vi "S1500_S7Com_W+R_Loop.vi"() -> ()   [LabVIEW 2018]
doc: "Demonstrates Reading from and Writing to a PLC in a loop."
uses:
  S7Com_Source_inkl_IP/S7Com_PLC_Data.ctl
  S1500_S7Com_Data_Array.ctl
  S1500_S7Com_RW_CMD.ctl
  S1500_S7Com_Address_Area.ctl
  S1500_S7Com_Start_Add.ctl
  S1500_S7Com_Transport_Size.ctl
  S1500_S7Com_Function.ctl
  S7Com_Source_inkl_IP/S7Com_Function.ctl
  S7Com_Source_inkl_IP/S7Com_Transport_Size.ctl
  S7Com_Source_inkl_IP/S7Com_Address_Area.ctl
  S7Com_Source_inkl_IP/S7Com_Start_Add.ctl
  S7Com_Source_inkl_IP/S7Com_RW_CMD.ctl
panel:
  out "x+1":u32
  out "Read_Data 2":T1
  in  "RW_CMD":T2={"Read Length"=1, "Data Block #"=1, "S7_Add_Area"=132, "Start Address"=0, "S7_Transport_Size"=5, "S7_Function"=2, "IP-Address"=""} {"S7_Function" items=["Read"=4, "Write"=5]; "S7_Transport_Size" items=["BIT"=1, "BYTE"=2, "CHAR"=3, "WORD"=4, "INT"=5, "DWORD"=6, "DINT"=7, "REAL"=8]; "S7_Add_Area" items=["P Area"=128, "I Area"=129, "O Area"=130, "M Area"=131, "DB Area"=132, "Counter"=40, "Timer"=41]}
  out "Read_Data":T1
  out "Loops":u32
  out "Data from PLC":T7
  in  "Data to PLC":T7
  out "Write Error":bool
  out "Read Error":bool=TRUE
  in  "wait":u32=1000 min=500 step=1
  in  "stop":bool
  in  "timeout ms":i32=5000
  in  "PLC IP Address":string="192.168.84.1"
  out "error out":errorcluster={"status"=TRUE, "code"=59, "source"="LIB_PLC_communication.lvlib:S1500_S7Com_OPEN(SubVI).vi:6290002->LIB_PLC_communication.lvlib:S1500_S7Com_W+R_Loop.vi中的打开TCP连接"}
  in  "error in (no error)":errorcluster
  # "DB-12, Write to PLC"
  # "DB-11, Read from PLC"
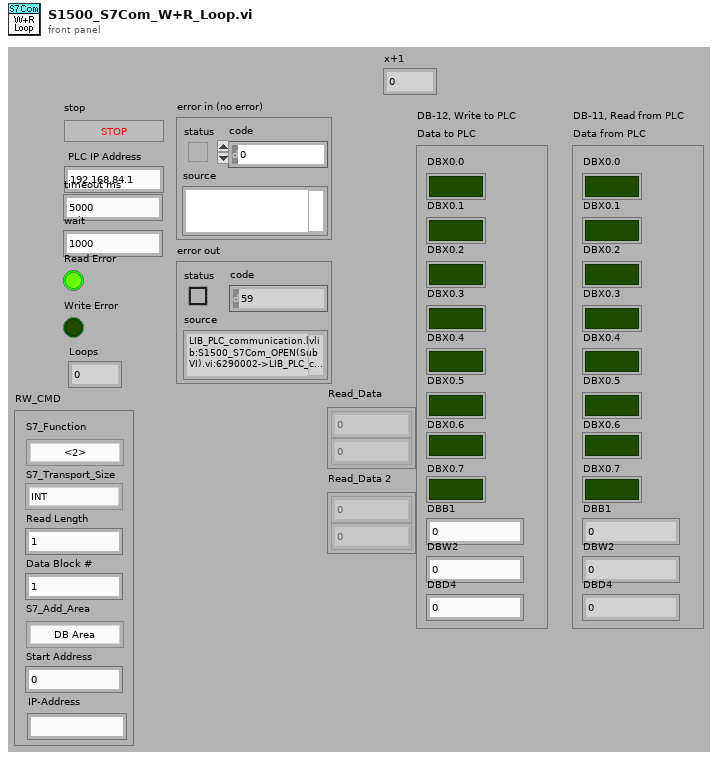
[diagram p1: front panel]
types:
  T1 = typedef "S1500_S7Com_Data_Array.ctl" = i32[]
  T2 = typedef "S1500_S7Com_RW_CMD.ctl" = cluster{"Read Length":u16, "Data Block #":u16, "S7_Add_Area":T3, "Start Address":T4, "S7_Transport_Size":T5, "S7_Function":T6, "IP-Address":string}
  T3 = typedef "S1500_S7Com_Address_Area.ctl" = u8
  T4 = typedef "S1500_S7Com_Start_Add.ctl" = u16
  T5 = typedef "S1500_S7Com_Transport_Size.ctl" = u8
  T6 = typedef "S1500_S7Com_Function.ctl" = u8
  T7 = typedef "S7Com_PLC_Data.ctl" = cluster{"DBX0.0":bool, "DBX0.1":bool, "DBX0.2":bool, "DBX0.3":bool, "DBX0.4":bool, "DBX0.5":bool, "DBX0.6":bool, "DBX0.7":bool, "DBB1":i8, "DBW2":i16, "DBD4":i32}
  T8 = typedef "S7Com_RW_CMD.ctl" = cluster{"Read Length":u16, "Data Block #":u16, "S7_Add_Area":T9, "Start Address":T10, "S7_Transport_Size":T11, "S7_Function":T12, "IP-Address":string}
  T9 = typedef "S7Com_Address_Area.ctl" = u8
  T10 = typedef "S7Com_Start_Add.ctl" = u16
  T11 = typedef "S7Com_Transport_Size.ctl" = u8
  T12 = typedef "S7Com_Function.ctl" = u8
  T13 = typedef "S7Com_Data_Array.ctl" = i32[]
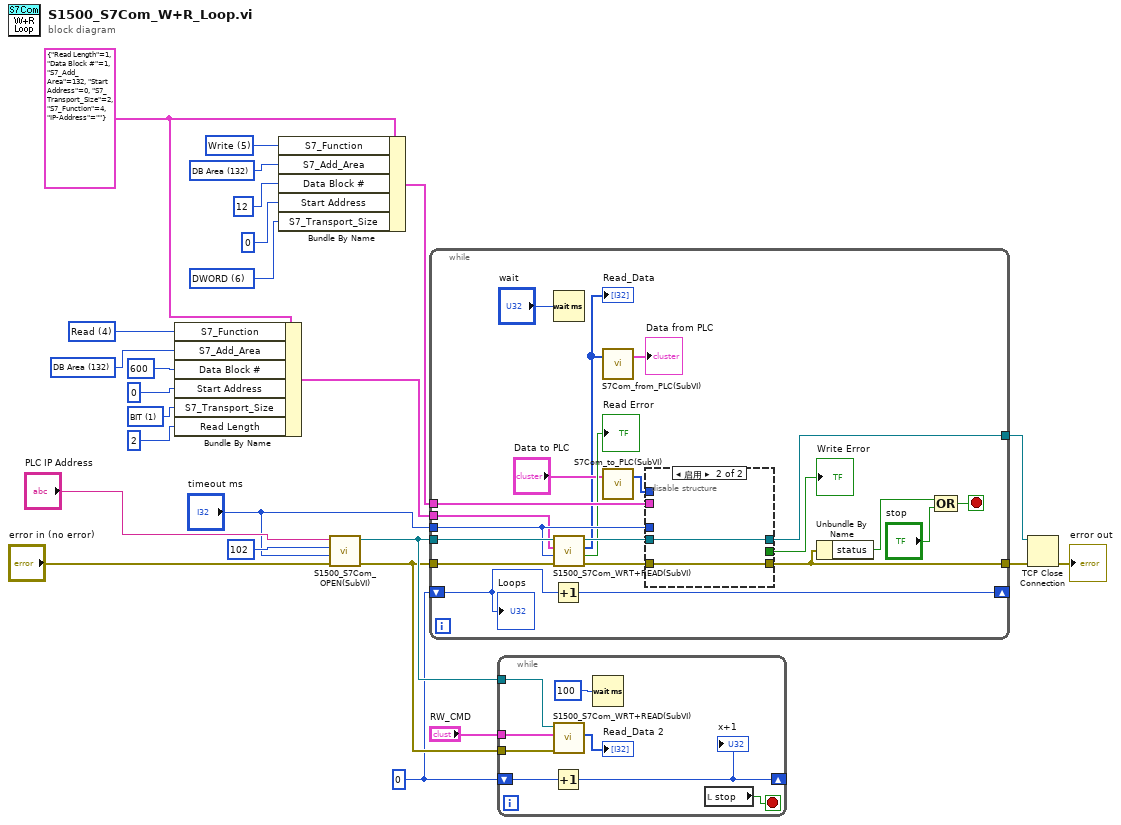
[diagram p0: block diagram]
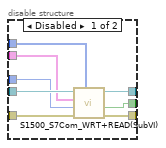
[diagram p2: hidden frame]
diagram:
  w1 = u32 0
  w7 = T8 {"Read Length"=1, "Data Block #"=1, "S7_Add_Area"=132, "Start Address"=0, "S7_Transport_Size"=2, "S7_Function"=4, "IP-Address"=""} ("RW_CMD")
  w8 = T11 6 items=["BIT"=1, "BYTE"=2, "CHAR"=3, "WORD"=4, "INT"=5, "DWORD"=6, "DINT"=7, "REAL"=8] ("S7_Transport_Size")
  w11 = T9 132 items=["P Area"=128, "I Area"=129, "O Area"=130, "M Area"=131, "DB Area"=132, "Counter"=40, "Timer"=41] ("S7_Add_Area")
  w12 = T12 5 items=["Read"=4, "Write"=5] ("S7_Function")
  w13 = T11 1 items=["BIT"=1, "BYTE"=2, "CHAR"=3, "WORD"=4, "INT"=5, "DWORD"=6, "DINT"=7, "REAL"=8] ("S7_Transport_Size")
  w16 = T9 132 items=["P Area"=128, "I Area"=129, "O Area"=130, "M Area"=131, "DB Area"=132, "Counter"=40, "Timer"=41] ("S7_Add_Area")
  w17 = T12 4 items=["Read"=4, "Write"=5] ("S7_Function")
  n1 = Bundle By Name(cluster=w7, "S7_Function"=w17, "S7_Add_Area"=w16, "Data Block #"=u16 600, "Start Address"=T10 0, "S7_Transport_Size"=w13, "Read Length"=u16 2) -> (w18:T8)
  n2 = Bundle By Name(cluster=w7, "S7_Function"=w12, "S7_Add_Area"=w11, "Data Block #"=u16 12, "Start Address"=T10 0, "S7_Transport_Size"=w8) -> (w5:T8)
  n3 = call "S1500_S7Com_OPEN(SubVI).vi"("remote address"="PLC IP Address", "remote port"=u16 102, "timeout ms"="timeout ms", "error in (no error)"="error in (no error)") -> ("connection ID out"=w4:refnum<k5>, "error out"=w3:errorcluster)  [unwired: 3 out]
  n4 = while {
    tunnel: w4 -> [w46]
    tunnel: [w42] -> w21
    tunnel: [w32] -> w20
    tunnel: w3 -> [w45]
    tunnel: "timeout ms" -> [w40]
    tunnel: w18 -> [w36]
    tunnel: w5 -> [w35]
    shift-right: [w27] -> _
    shift-left: w1 -> [w26]
    stop <- w38 stop-if-true
    n5 = Increment(x=w26) -> (x+1=w27:u32)
    n6 = Wait (ms)(milliseconds to wait="wait") -> ()  [unwired: 1 out]
    n7 = call "S1500_S7Com_WRT+READ(SubVI).vi"("error in"=w45, "timeout ms (25000)"=w40, "RW_CMD"=w36, "connection ID in"=w46) -> ("error out"=w41:errorcluster, "Error"=→"Read Error":bool, "Read_Data"=w28:T1, "connection ID out"=w43:refnum<k5>)  [unwired: 1 in]
    "Read_Data" <- w28
    n8 = call "S7Com_from_PLC(SubVI).vi"("S7Com_Data_Array_In"=w28) -> ("from_PLC_Out"=→"Data from PLC":T7)  [unwired: 2 out]
    n9 = call "S7Com_to_PLC(SubVI).vi"("to_PLC_In"="Data to PLC") -> ("S7Com_Data_Array_Out"=w31:T13)  [unwired: 2 out]
    n10 = disable-structure shown="启用" {
      disable-tunnel: w43 -> [w54 w56]
      disable-tunnel: [w53 w56] -> w42
      disable-tunnel: w41 -> [w52 w55]
      disable-tunnel: w40 -> [w51 _]
      disable-tunnel: w35 -> [w50 _]
      disable-tunnel: [w49 _] -> w33
      disable-tunnel: [w48 w55] -> w32
      disable-tunnel: w31 -> [w47 _]
      frame Disabled {
        n11 = call "S1500_S7Com_WRT+READ(SubVI).vi"("Write_Data"=w47, "error in"=w52, "timeout ms (25000)"=w51, "RW_CMD"=w50, "connection ID in"=w54) -> ("error out"=w48:errorcluster, "Error"=w49:bool, "connection ID out"=w53:refnum<k5>)  [unwired: 1 out]
      }
      frame Enabled {
      }
    }
    "Write Error" <- w33
    n12 = Unbundle By Name(w32) -> ("status"=w37:bool)
    n13 = Compound Arithmetic op=OR(w37, "stop") -> (w38:bool)
    "Loops" <- w26
  }
  n14 = while {
    tunnel: w4 -> [w64]
    tunnel: w3 -> [w63]
    tunnel: "RW_CMD" -> [w62]
    shift-right: [w58] -> _
    shift-left: w1 -> [w57]
    stop <- w60 stop-if-true
    n15 = Increment(x=w57) -> (x+1=w58:u32)
    "x+1" <- w58
    n16 = call "S1500_S7Com_WRT+READ(SubVI).vi"("error in"=w63, "RW_CMD"=w62, "connection ID in"=w64) -> ("Read_Data"=→"Read_Data 2":T1)  [unwired: 2 in, 3 out]
    n17 = Wait (ms)(milliseconds to wait=100) -> ()  [unwired: 1 out]
    n18 = local read "stop"() -> (w60:bool)
  }
  n19 = TCP Close Connection(connection ID=w21, error in (no error)=w20) -> (error out=→"error out":errorcluster)  [unwired: 2 out]
